vi "proc cal image-make bandpass.vi"(1 "HIGH bandpass\n(mode)":sgl format="%.2f", 2 "LOW bandpass\n(mode)":sgl format="%.2f", 3 "# of points (cross size)":i32) -> (0 "Cosine bandpass":sgl[](array[numeric]) format="%.2e")   [LabVIEW 2014]
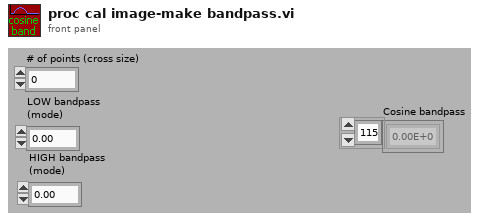
[diagram p1: front panel]
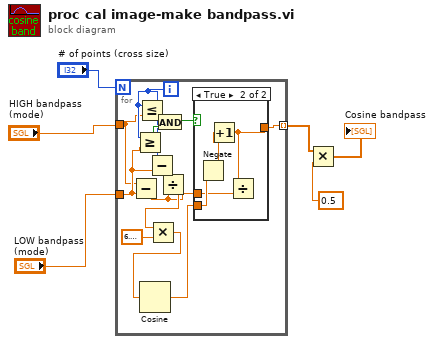
[diagram p0: block diagram]
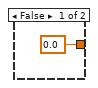
[diagram p2: hidden frame]
diagram:
  n1 = for {
    N: "# of points (cross size)" -> [_]
    tunnel: [w16] -> w3 mode=indexing
    tunnel: "LOW bandpass\n(mode)" -> [w9]
    tunnel: "HIGH bandpass\n(mode)" -> [w8]
    i -> [w10]
    n2 = Subtract(x=w8, y=w9) -> (x-y=w7:sgl)
    n3 = Greater Or Equal?(x=w10, y=w9) -> (x >= y?=w19:bool)
    n4 = Less Or Equal?(x=w10, y=w8) -> (x <= y?=w17:bool)
    n5 = Subtract(x=w10, y=w9) -> (x-y=w15:sgl)
    n6 = And(x=w17, y=w19) -> (x .and. y?=w18:bool)
    n7 = Divide(x=w15, y=w7) -> (x/y=w14:sgl)
    n8 = Multiply(x=w14, y=sgl 6.2831855) -> (x*y=w12:sgl)
    n9 = Cosine(x=w12) -> (cos(x)=w11:sgl)
    n10 = case shown="True" w18 {
      tunnel: [sgl 0.0 w22] -> w16
      tunnel: w11 -> [_ w24]
      tunnel: w7 -> [_ w21]
      frame False {
      }
      frame True {
        n11 = Negate(x=w24) -> (-x=w23:sgl)
        n12 = Increment(x=w23) -> (x+1=w22:sgl)
        n13 = Divide(x=w22, y=w21) -> ()  [unwired: 1 out]
      }
    }
  }
  n14 = Multiply(x=w3, y=sgl 0.5) -> (x*y=→"Cosine bandpass":sgl[])
